vi "Read DBL.vi"(8 "error in (no error)":errorcluster, 9 "element data type":dbl, 10 "Tag Name":string, 11 "Current Value Table in":refnum<class "Current Value Table.lvclass">) -> (0 "error out":errorcluster, 2 "value":dbl, 3 "Current Value Table out":refnum<class "Current Value Table.lvclass">)   [LabVIEW 2024, in "Current Value Table.lvlib" / "Current Value Table.lvclass"]
uses:
  Current Value Table.lvclass
  CVT_DBL/CVT_DBL.lvclass
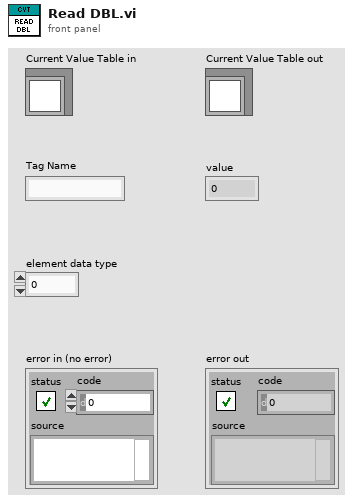
[diagram p1: front panel]
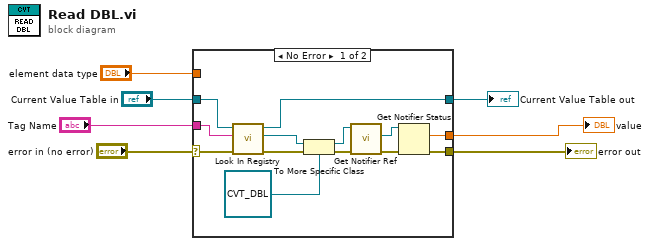
[diagram p0: block diagram]
diagram:
  n1 = case shown="No Error" "error in (no error)" {
    selector: "error in (no error)" -> [w14 w22]
    tunnel: [w8 w22] -> w6
    tunnel: [w19 w21] -> w4
    tunnel: "Current Value Table in" -> [w20 w21]
    tunnel: "Tag Name" -> [w17 _]
    tunnel: "element data type" -> [_ _]
    tunnel: [w9 _] -> w1
    frame No Error {
      n2 = call-dynamic "Look In Registry.vi"("error in (no error)"=w14, "Tag Name"=w17, "Current Value Table in"=w20) -> ("error out"=w15:errorcluster, "CVT_Item out"=w18:refnum<class "iCVT_Item.lvclass">, "Current Value Table out"=w19:refnum<class "Current Value Table.lvclass">)  [unwired: 5 in, 1 out]
      n3 = To More Specific Class(target class=refnum<class "CVT_DBL.lvclass"> refnum ("Current Value Table.lvlib:CVT_DBL.lvclass"), reference=w18, error in=w15) -> (specific class reference=w12:refnum<class "CVT_DBL.lvclass">, error out=w11:errorcluster)
      n4 = call-dynamic "Get Notifier Ref.vi"("error in (no error)"=w11, "CVT_DBL in"=w12) -> ("error out"=w10:errorcluster, "notifier out"=w13:refnum<notifier>)  [unwired: 7 in, 1 out]
      n5 = Get Notifier Status(notifier=w13, error in (no error)=w10) -> (current notification=w9:dbl, error out=w8:errorcluster)  [unwired: 3 out]
    }
    frame Error {
    }
  }
  "error out" <- w6
  "Current Value Table out" <- w4
  "value" <- w1
